vi "Create.vi"(8 "error in (no error)":errorcluster, 10 "Input":string) -> (0 "error out":errorcluster, 3 "Proto":refnum<class "Proto.lvclass">)   [LabVIEW 2021, in "Proto.lvclass"]
uses:
  Proto.lvclass
  Proto.lvclass/Proto.ctl
  Helpers/Helpers.lvlib
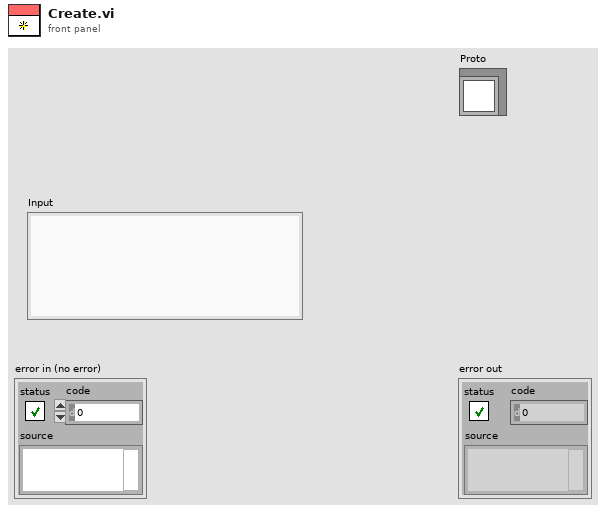
[diagram p1: front panel]
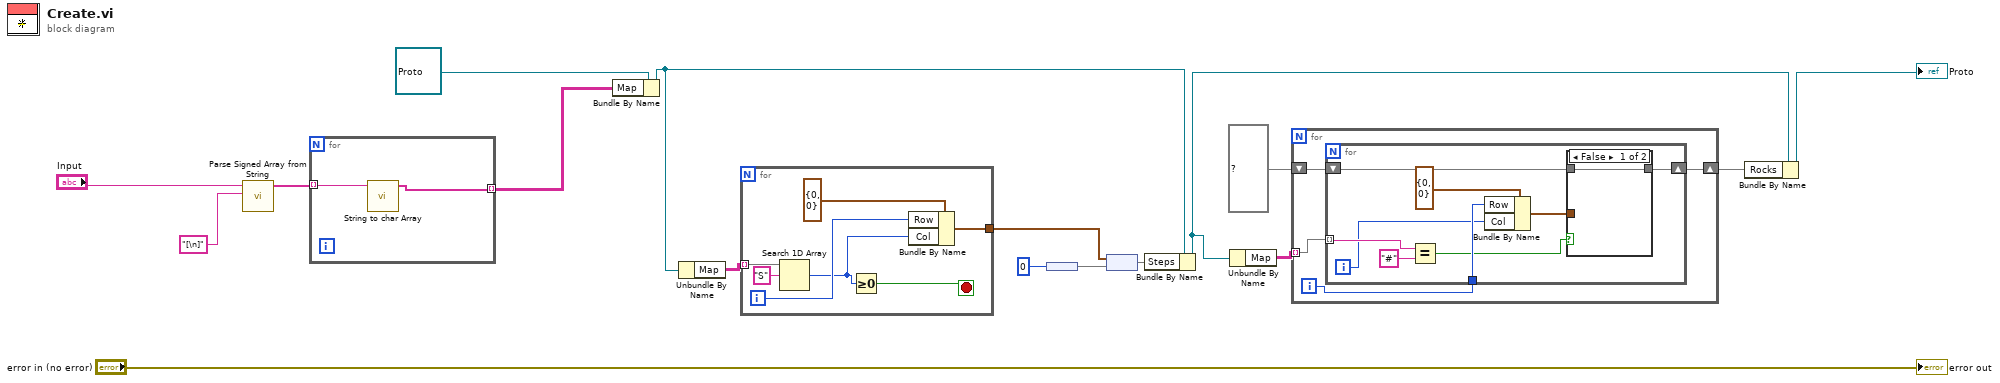
[diagram p0: block diagram]
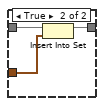
[diagram p2: hidden frame]
diagram:
  n1 = call "Parse Signed Array from String.vi"("Delimiter regex"="[\n]", "Input"="Input") -> ("Parsed Array"=w13:string[])  [unwired: 8 in, 1 out]
  n2 = for {
    tunnel: w13 -> [w19] mode=indexing
    tunnel: [w18] -> w12 mode=indexing
    n3 = call "String to char Array.vi"("Row"=w19) -> ("Array"=w18:string[])  [unwired: 10 in]
  }
  n4 = Bundle By Name(cluster=refnum<class "Proto.lvclass"> refnum ("Proto"), "Map"=w12) -> (w10:refnum<class "Proto.lvclass">)
  n5 = Unbundle By Name(w10) -> ("Map"=w11:string[][])
  n6 = for {
    tunnel: w11 -> [w26] mode=indexing
    tunnel: [w20] -> w7
    i -> [w22]
    stop <- w24 stop-if-true
    n7 = Search 1D Array(1D array=w26, element="S") -> (index of element=w21:i32)  [unwired: 1 in]
    n8 = Greater Or Equal To 0?(x=w21) -> (x >= 0?=w24:bool)
    n9 = Bundle By Name(cluster=cluster{"Row":i32, "Col":i32} {"Row"=0, "Col"=0} ("Coord"), "Row"=w22, "Col"=w21) -> (w20:cluster{"Row":i32, "Col":i32})
  }
  n10 = node(0 ("index of element")) -> (w8:set{i32})
  n11 = node(w7, w8) -> (w6:map{cluster{"Row":i32, "Col":i32}, set{i32}})
  n12 = Bundle By Name(cluster=w10, "Steps"=w6) -> (w4:refnum<class "Proto.lvclass">)
  n13 = Unbundle By Name(w4) -> ("Map"=w5:string[][])
  n14 = for {
    tunnel: w5 -> [w30] mode=indexing
    shift-right: [w27] -> w1
    shift-left: set{cluster{"Row":i32, "Col":i32}} {} ("set") -> [w28]
    i -> [w29]
    n15 = for {
      tunnel: w30 -> [w38] mode=indexing
      tunnel: w29 -> [w36]
      shift-right: [w33] -> w27
      shift-left: w28 -> [w34]
      i -> [w35]
      n16 = Equal?(x=w38, y="#") -> (x = y?=w32:bool)
      n17 = Bundle By Name(cluster=cluster{"Row":i32, "Col":i32} {"Row"=0, "Col"=0} ("Coord"), "Row"=w36, "Col"=w35) -> (w31:cluster{"Row":i32, "Col":i32})
      n18 = case shown="False" w32 {
        tunnel: w34 -> [w40 w43]
        tunnel: [w40 w42] -> w33
        tunnel: w31 -> [_ w41]
        frame False {
        }
        frame True {
          n19 = Insert Into Set(10:w41, 11:w43) -> (3:w42:set{cluster{"Row":i32, "Col":i32}})  [unwired: 1 out]
        }
      }
    }
  }
  n20 = Bundle By Name(cluster=w4, "Rocks"=w1) -> (→"Proto":refnum<class "Proto.lvclass">)
  "error out" <- "error in (no error)"
